vi "Abs Encoder Invert(SubVI).vi"(7 "Sensor Phase":bool, 11 "encoder":i32) -> (3 "encoder reversed":i32)   [LabVIEW 2018, in "Elevator.lvlib" / "Elevator Linear.lvclass"]
doc: "This VI inverts the encoder for the Elevator."
uses:
  Elevator Linear.lvclass
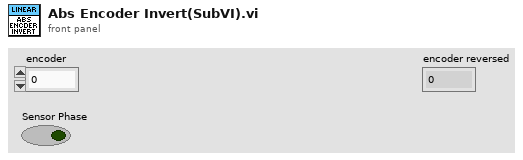
[diagram p1: front panel]
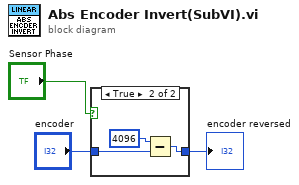
[diagram p0: block diagram]
diagram:
  n1 = case shown="True" "Sensor Phase" {
    tunnel: "encoder" -> [w4 w7]
    tunnel: [w4 w6] -> w1
    frame False {
    }
    frame True {
      n2 = Subtract(x=4096, y=w7) -> (x-y=w6:i32)
    }
  }
  "encoder reversed" <- w1
